vi "是否可下.vi"(0 "当前棋盘状态":i32[][](array[numeric]), 7 "行":sgl, 9 "列":i16) -> (4 "当前棋盘状态":i32[][](array[numeric]), 8 "行":sgl, 10 "列":i16, 15 "当前点可下?":bool)   [LabVIEW 2018]
panel:
  # "0"
  # "1"
  # "2"
  # "3"
  # "4"
  # "5"
  # "6"
  # "7"
  # "8"
  # "9"
  # "10"
  # "11"
  # "12"
  # "13"
  # "14"
  # "0"
  # "1"
  # "2"
  # "3"
  # "4"
  # "5"
  # "6"
  # "7"
  # "8"
  # "9"
  # "10"
  # "11"
  # "12"
  # "13"
  # "14"
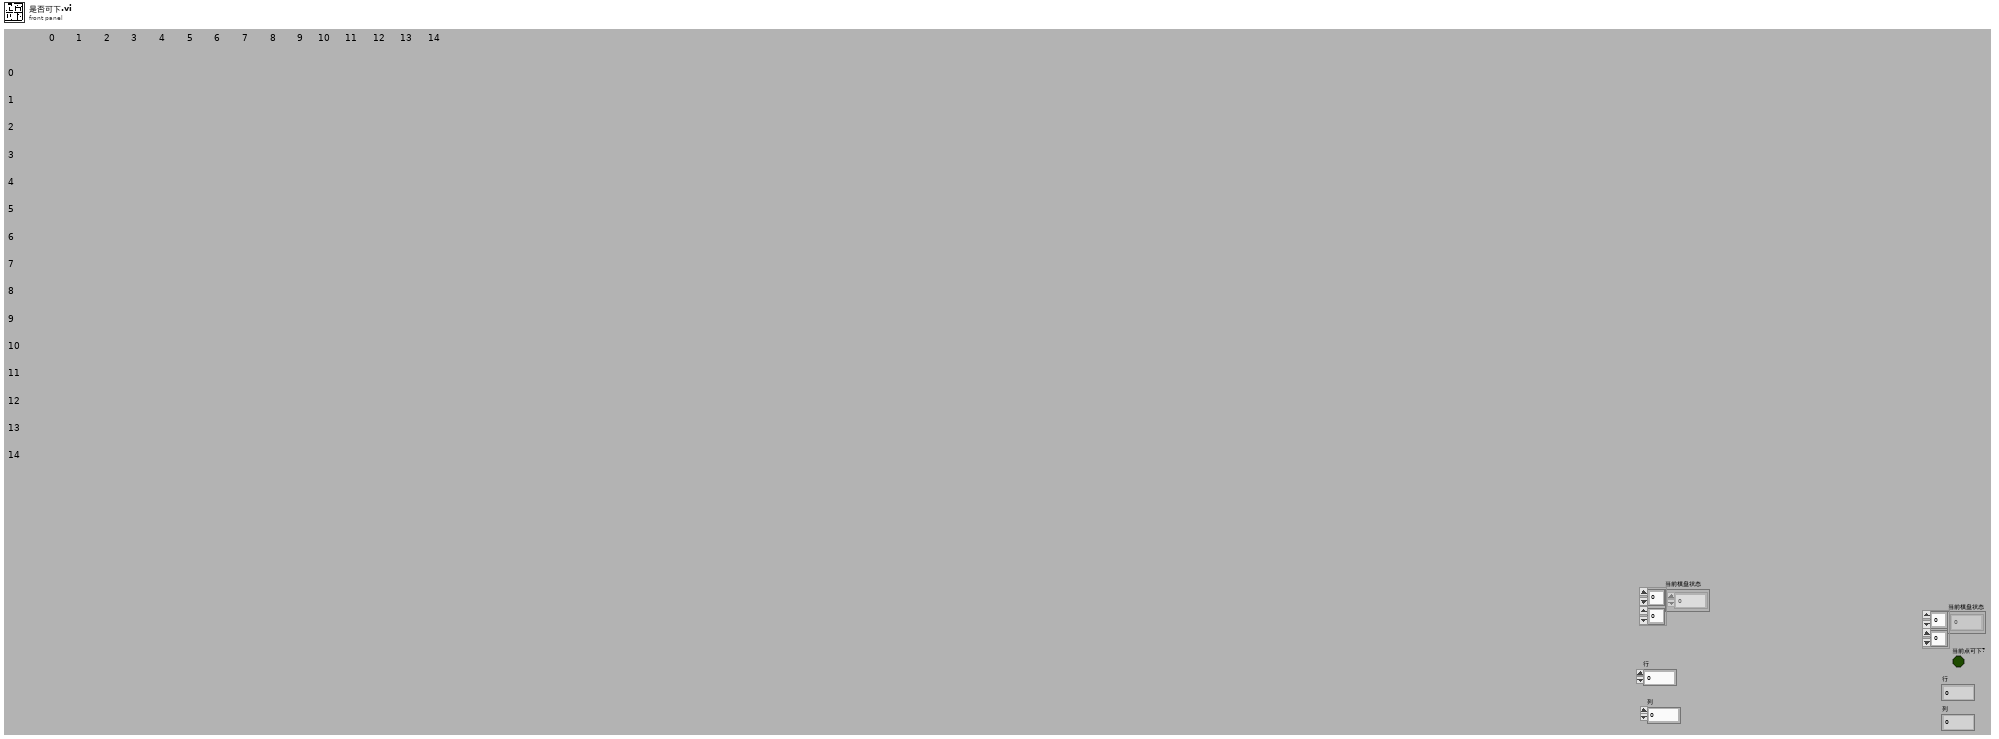
[diagram p1: front panel]
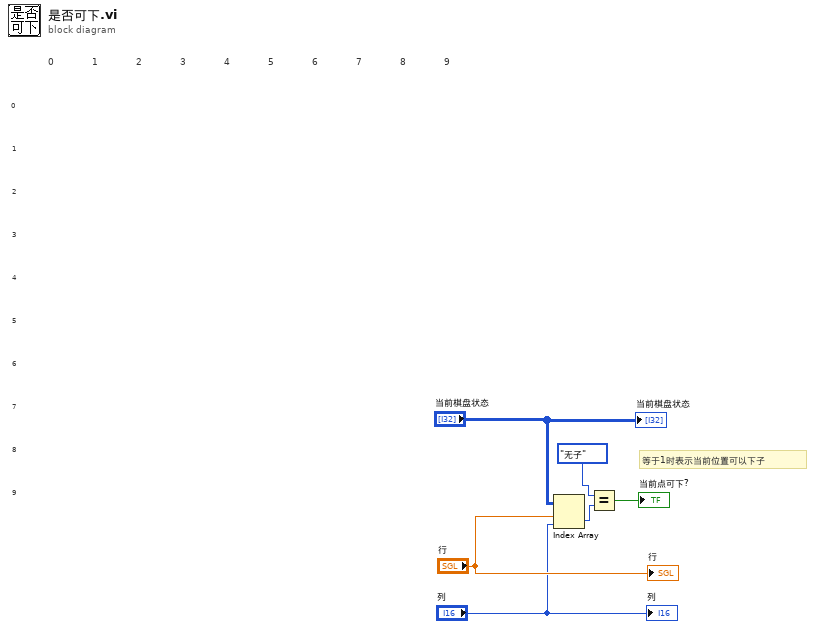
[diagram p0: block diagram]
diagram:
  # "等于1时表示当前位置可以下子"
  # "9"
  # "8"
  # "7"
  # "6"
  # "5"
  # "4"
  # "3"
  # "2"
  # "1"
  # "0"
  # "9"
  # "8"
  # "7"
  # "6"
  # "5"
  # "4"
  # "3"
  # "2"
  # "1"
  # "0"
  n1 = Index Array(array="当前棋盘状态", index (row)="行", index (col)="列") -> (element=w6:i32)
  n2 = Equal?(x=enum16{"白子", "无子", "黑子"}."无子", y=w6) -> (x = y?=→"当前点可下?":bool)
  "当前棋盘状态" <- "当前棋盘状态"
  "行" <- "行"
  "列" <- "列"
